vi "Downsample 1D array.vi"(10 "Ave N":dbl, 11 "Arrray In":dbl[](array[numeric])) -> (3 "Array Out":dbl[](array[numeric]))   [LabVIEW 2016]
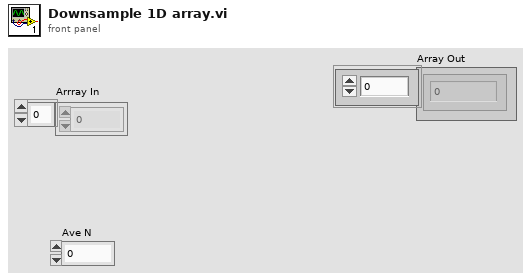
[diagram p1: front panel]
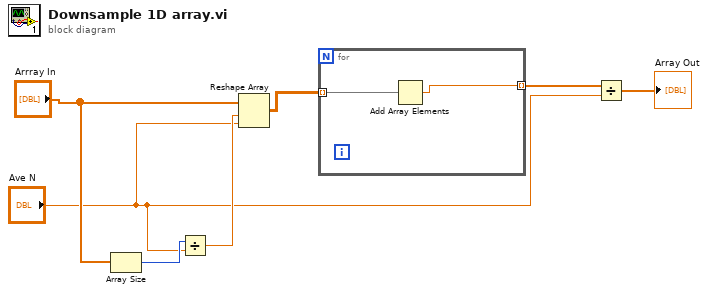
[diagram p0: block diagram]
diagram:
  n1 = Array Size(array="Arrray In") -> (size(s)=w6:i32)
  n2 = Divide(x=w6, y="Ave N") -> (x/y=w5:dbl)
  n3 = Reshape Array("Arrray In", w5, "Ave N") -> (w4:dbl[][])
  n4 = for {
    tunnel: w4 -> [w9] mode=indexing
    tunnel: [w8] -> w3 mode=indexing
    n5 = Add Array Elements(numeric array=w9) -> (sum=w8:dbl)
  }
  n6 = Divide(x=w3, y="Ave N") -> (x/y=→"Array Out":dbl[])
